vi "BuildArray.vi"(1 "Columns":i32, 2 "Rows":i32, 3 "Array":dbl[](array[numeric])) -> (0 "output array":dbl[][](array[numeric]))   [LabVIEW 2013]
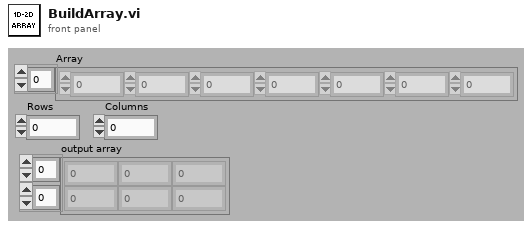
[diagram p1: front panel]
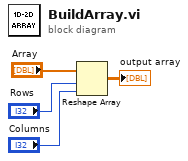
[diagram p0: block diagram]
diagram:
  n1 = Reshape Array("Array", "Rows", "Columns") -> (→"output array":dbl[][])
